vi "Fire Update Event.vi"(8 "error in (no error)":errorcluster, 10 "Force (F)":bool, 11 "Terminal in":refnum<class "Terminal.lvclass">) -> (0 "error out":errorcluster, 3 "Terminal out":refnum<class "Terminal.lvclass">)   [LabVIEW 2020, in "Terminal.lvlib" / "Terminal.lvclass"]
uses:
  Terminal.lvclass
  Terminal.lvclass/Terminal.ctl
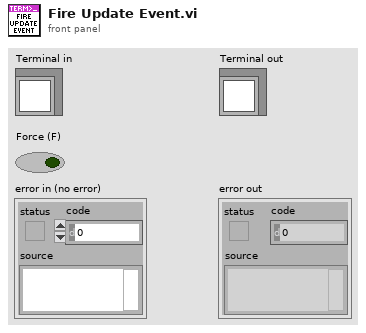
[diagram p1: front panel]
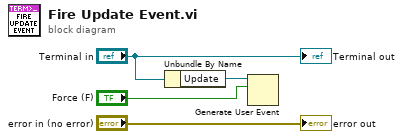
[diagram p0: block diagram]
diagram:
  n1 = Unbundle By Name("Terminal in") -> ("Update"=w1:refnum<user-event>)
  n2 = Generate User Event(user event=w1, event data cluster="Force (F)") -> ()  [unwired: 2 in, 2 out]
  "error out" <- "error in (no error)"
  "Terminal out" <- "Terminal in"
